vi "Create Device.vi"() -> ()   [LabVIEW 2019]
uses:
  E:/UPWORK/NTU-APR-LAB/photonics-measurements-tool-labview/project/data/Thorlabs.MotionControl.Controls.dll
  data/Thorlabs.MotionControl.Controls.dll
panel:
  out "CloseDevice":bool
  out "error out":errorcluster
  out "CreateDevice":bool
  in  "KCubeInertialMotorControl":refnum<k24>(container)
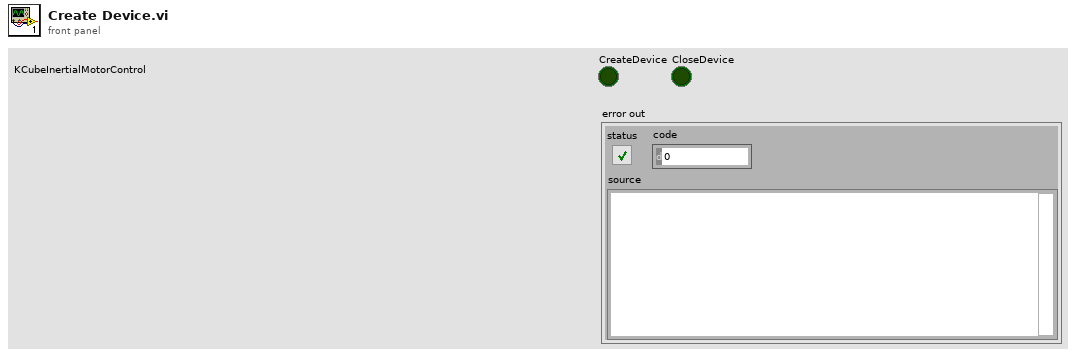
[diagram p1: front panel]
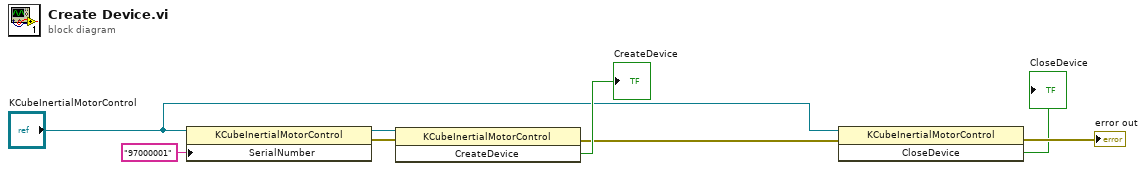
[diagram p0: block diagram]
diagram:
  n1 = property class="KCubeInertialMotorControl"(reference="KCubeInertialMotorControl", "SerialNumber"="97000001") -> (reference out=w7:refnum<k24>, error out=w6:errorcluster)  [unwired: 1 in]
  n2 = invoke class="KCubeInertialMotorControl" method="CreateDevice"(reference=w7, error in=w6) -> (error out=w3:errorcluster, "CreateDevice"=→"CreateDevice":bool)  [unwired: 1 in, 1 out]
  n3 = invoke class="KCubeInertialMotorControl" method="CloseDevice"(reference="KCubeInertialMotorControl", error in=w3) -> (error out=→"error out":errorcluster, "CloseDevice"=→"CloseDevice":bool)  [unwired: 1 in, 1 out]
